vi "CODCrMB_api.vi"(6 "Slave ID":u8=1, 7 "STEP":enum16{"open", "read", "write", "close"}(ring)=enum."read", 8 "Error in":errorcluster caption="Error in (no error)", 9 "values":u16[](array[numeric]), 10 "quantity":u16, 11 "starting address":u16 format="%04xH") -> (0 "error out":errorcluster, 1 "MB session out":refnum<class "MB_Master.lvclass">, 2 "MB_TCP session":refnum<class "MB_Master_TCP.lvclass">, 3 "Registers":u16[](array[numeric]))   [LabVIEW 2016, in "CODCr库.lvlib"]
uses:
  <vilib>/Plasmionique/MB Master/MB_Master/MB_Master.lvclass
  <vilib>/Plasmionique/MB Master/MB_Master_TCP/MB_Master_TCP.lvclass
  D:/Program Files (x86)/National Instruments/LabVIEW 2016/vi.lib/Plasmionique/MB Master/MB_Master/MB_Master.lvclass
  <vilib>/Plasmionique/MB Master/MB_Master_Serial/MB_Master_Serial.lvclass
  <vilib>/Plasmionique/MB Master/MB Master.lvlib
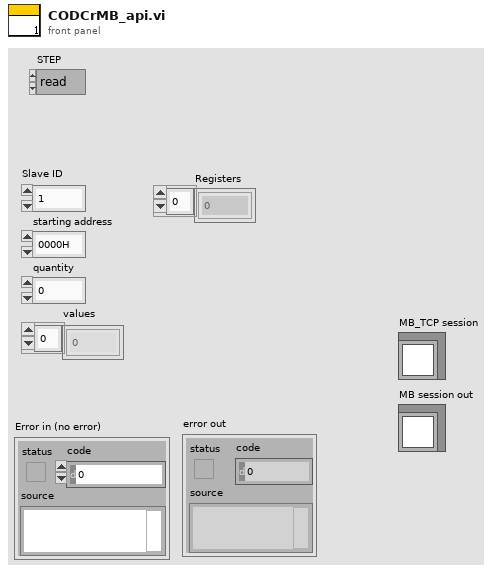
[diagram p1: front panel]
types:
  T1 = cluster{"baud rate (bps)":u32, "stop bits":u16, "parity":u16, "flow control":u16, "timeout":u32, "retries":i32}
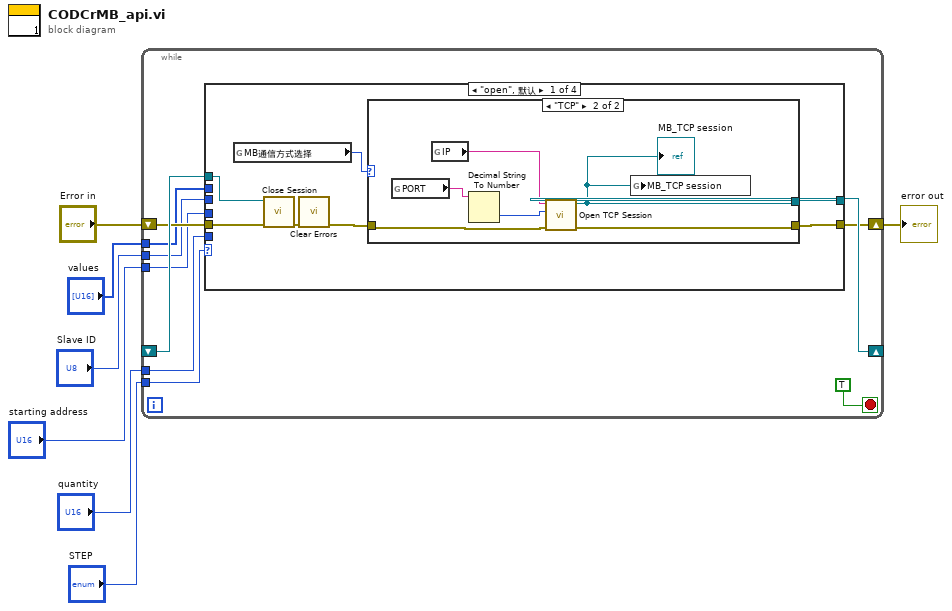
[diagram p0: block diagram]
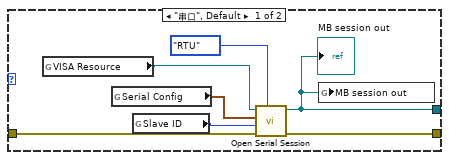
[diagram p2: hidden frame]
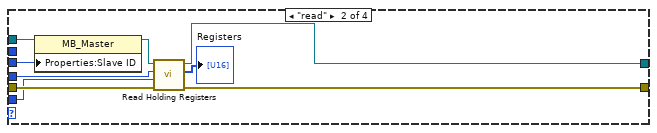
[diagram p3: hidden frame]
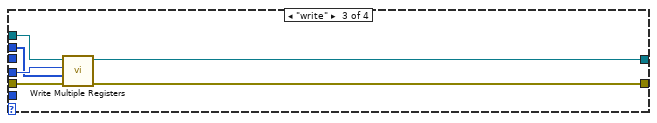
[diagram p4: hidden frame]
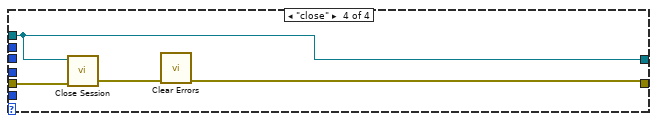
[diagram p5: hidden frame]
diagram:
  n1 = while {
    shift-right: [w9] -> _
    shift-left: _ -> [w17]
    shift-right: [w8] -> w6
    shift-left: "Error in" -> [w16]
    tunnel: "Slave ID" -> [w15]
    tunnel: "starting address" -> [w14]
    tunnel: "quantity" -> [w13]
    tunnel: "STEP" -> [w12]
    tunnel: "values" -> [w11]
    stop <- TRUE stop-if-true
    n2 = case shown="\"open\", 默认" w12 {
      tunnel: w17 -> [w22 w39 w50 w55]
      tunnel: w16 -> [w21 w46 w52 w56]
      tunnel: [w23 w45 w49 w55] -> w9
      tunnel: [w24 w44 w51 w53] -> w8
      tunnel: w15 -> [_ w42 _ _]
      tunnel: w14 -> [_ w41 w48 _]
      tunnel: w13 -> [_ w40 _ _]
      tunnel: w11 -> [_ _ w47 _]
      frame "open", Default {
        n3 = global read "CODcr全局变量.vi" "MB通信方式选择"() -> (w18:enum16{"串口", "TCP"})
        n4 = call-dynamic "Close Session.vi"("error in (no error)"=w21, "MB session in"=w22) -> ("error out"=w20:errorcluster)  [unwired: 9 in]
        n5 = call <vilib>:"Clear Errors.vi"("error in (no error)"=w20) -> ("error out"=w19:errorcluster)  [unwired: 5 in, 1 out]
        n6 = case shown="\"TCP\"" w18 {
          tunnel: [w30 w33] -> w24
          tunnel: [w25 w32] -> w23
          tunnel: w19 -> [w29 w34]
          frame "串口", Default {
            n7 = global read "CODcr全局变量.vi" "VISA Resource"() -> (w27:refnum<visa-resource-name>)
            n8 = global read "CODcr全局变量.vi" "Serial Config"() -> (w28:T1)
            n9 = global read "CODcr全局变量.vi" "Slave ID"() -> (w26:u8)
            n10 = call <vilib>:"Open Serial Session.vi"("Mode (RTU)"=enum16{"RTU", "ASCII"}."RTU", "Error in"=w29, "Slave ID"=w26, "Serial Config"=w28, "VISA Resource"=w27) -> ("Error out"=w30:errorcluster, "MB_Serial session"=w25:refnum<class "MB_Master_Serial.lvclass">)  [unwired: 5 in]
            "MB session out" <- w25
            n11 = global write "CODcr全局变量.vi" "MB session out"(w25) -> ()
          }
          frame "TCP" {
            n12 = global read "CODcr全局变量.vi" "PORT"() -> (w37:string)
            n13 = global read "CODcr全局变量.vi" "IP"() -> (w36:string)
            n14 = Decimal String To Number(string=w37) -> (number=w35:i32)  [unwired: 2 in, 1 out]
            n15 = call <vilib>:"Open TCP Session.vi"("error in (no error)"=w34, "Port (502)"=w35, "IP Address"=w36) -> ("error out"=w33:errorcluster, "MB_TCP session"=w32:refnum<class "MB_Master_TCP.lvclass">)  [unwired: 7 in]
            "MB_TCP session" <- w32
            n16 = global write "CODcr全局变量.vi" "MB_TCP session"(w32) -> ()
          }
        }
      }
      frame "read" {
        n17 = property class="MB_Master"(reference=w39, "Properties:Slave ID"=w42) -> (reference out=w38:refnum<class "MB_Master.lvclass">)  [unwired: 1 in, 1 out]
        n18 = call <vilib>:"Read Holding Registers.vi"("error in (no error)"=w46, "quantity"=w40, "starting address"=w41, "MB session in"=w38) -> ("error out"=w44:errorcluster, "Registers"=→"Registers":u16[], "MB session out"=w45:refnum<class "MB_Master.lvclass">)  [unwired: 5 in]
      }
      frame "write" {
        n19 = call <vilib>:"Write Multiple Registers.vi"("error in (no error)"=w52, "values"=w47, "starting address"=w48, "MB session in"=w50) -> ("error out"=w51:errorcluster, "MB session out"=w49:refnum<class "MB_Master.lvclass">)  [unwired: 6 in]
      }
      frame "close" {
        n20 = call-dynamic "Close Session.vi"("error in (no error)"=w56, "MB session in"=w55) -> ("error out"=w54:errorcluster)  [unwired: 9 in]
        n21 = call <vilib>:"Clear Errors.vi"("error in (no error)"=w54) -> ("error out"=w53:errorcluster)  [unwired: 5 in, 1 out]
      }
    }
  }
  "error out" <- w6
